vi "sc_setstep.vi"(8 "error in":errorcluster, 10 "step distance (steps)":dbl format="%#_13g", 11 "VISA in":refnum<visa-resource-name>) -> (0 "error out":errorcluster, 2 "Response":string, 3 "VISA out":refnum<visa-resource-name>)   [LabVIEW 2015]
uses:
  pipette cleaning/pressure box/cleaning_soft/controls/scientifica_commands.ctl
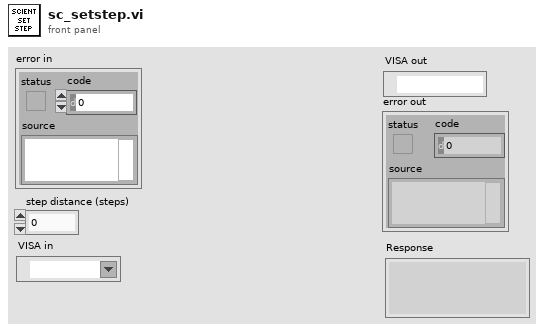
[diagram p1: front panel]
types:
  T1 = typedef "scientifica_commands.ctl" = enum16{"ANGLE", "INSET", "FIRST", "ZERO", "Pz", "P", "absz", "ACC", "TOP", "STOP", "rel", "relz", "abs", "IN", "vj", "APROACH", "OBJS", "OBJU", "OUT", "OBJ", "OBJL", "SET", "OBJD", "STEP", "SETSTEP", "S", "UUX", "UUY", "UUZ"}
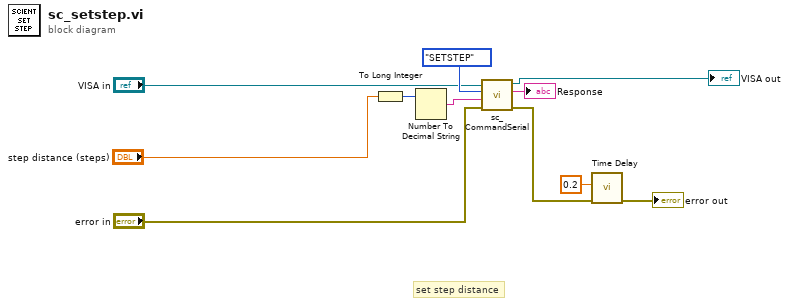
[diagram p0: block diagram]
diagram:
  # "set step distance"
  n1 = To Long Integer(number="step distance (steps)") -> (32bit integer=w10:i32)
  n2 = Number To Decimal String(number=w10) -> (decimal integer string=w9:string)  [unwired: 1 in]
  n3 = call "sc_CommandSerial.vi"("error in (no error)"="error in", "argument"=w9, "Scientifica commands"=scientifica_commands."SETSTEP", "VISA handle"="VISA in") -> ("error out"=w3:errorcluster, "Response"=→"Response":string, "Dup. VISA handle"=→"VISA out":refnum<visa-resource-name>)  [unwired: 4 in, 1 out]
  n4 = call "Time Delay"("error in (no error)"=w3, "Delay Time (s)"=0.2) -> ("error out"=→"error out":errorcluster)  [unwired: 9 in]
